vi "PathPlanner_Trajectory25_FindTimeForWaypointRelPos.vi"(9 "WaypointRelPos":dbl, 10 "AllWayPointRelPos":dbl[](array[numeric]), 11 "PathPlannerStates":T1[](array[typedef]) {"ModuleStates"."SWERVE_DRIVE_MODULE_STATE"."Angle"."SIN" format="%13.4f"; "ModuleStates"."SWERVE_DRIVE_MODULE_STATE"."Angle"."COS" format="%13.4f"; "ModuleStates"."SWERVE_DRIVE_MODULE_STATE"."Angle"."VALUE" format="%13.4f"; "ModuleStates"."FieldAngle"."SIN" format="%13.4f"; "ModuleStates"."FieldAngle"."COS" format="%13.4f"; "ModuleStates"."FieldAngle"."VALUE" format="%13.4f"; "ModuleStates"."FieldPos"."Y" format="%14.3f"; "ModuleStates"."FieldPos"."X" format="%14.3f"; "DeltaRot"."SIN" format="%13.4f"; "DeltaRot"."COS" format="%13.4f"; "DeltaRot"."VALUE" format="%13.4f"; "pose"."ROTATION"."SIN" format="%13.4f"; "pose"."ROTATION"."COS" format="%13.4f"; "pose"."ROTATION"."VALUE" format="%13.4f"; "pose"."TRANSLATION"."Y" format="%14.3f"; "pose"."TRANSLATION"."X" format="%14.3f"; "FieldSpeeds"."vOmega" format="%10.3f"; "FieldSpeeds"."vY" format="%10.3f"; "FieldSpeeds"."vX" format="%10.3f"; "Heading"."SIN" format="%13.4f"; "Heading"."COS" format="%13.4f"; "Heading"."VALUE" format="%13.4f"}) -> (3 "Time_Secs":dbl)   [LabVIEW 2019, in "PathPlanner24.lvlib"]
doc: "Find the time (seconds) for a particular waypoint relative position\n\nInputs:\n -- PathPlannerStates -- PathPlanner Trajectory States data cluster\n -- AllWaypointRelPos -- array of double - List of all waypoint relative positions.\n -- WaypointRelPos - double - The waypoint relative positon whose time is desired.\n\nOutputs:\n - Time_Secs - double - The trajectory time for this waypointRelPos."
uses:
  PathPlanner24.lvlib
  TypeDef/PathPlannerTrajectoryState25.ctl
  <vilib>/Rock Robotics/WPI/ThirdParty/JAS_Junk/TrajLib/TypeDef/ROTATION2D.ctl
  TypeDef/PathPlannerPathConstraints.ctl
  <vilib>/Rock Robotics/WPI/ThirdParty/JAS_Junk/TrajLib/TypeDef/CHASSIS_SPEEDS.ctl
  <vilib>/Rock Robotics/WPI/ThirdParty/JAS_Junk/TrajLib/TypeDef/POSE2D.ctl
  <vilib>/Rock Robotics/WPI/ThirdParty/JAS_Junk/TrajLib/TypeDef/TRANSLATION2D.ctl
  TypeDef/PathPlannerSwerveModTrajState.ctl
  <vilib>/Rock Robotics/WPI/ThirdParty/JAS_Junk/TrajLib/TypeDef/SWERVE_DRIVE_MODULE_STATE.ctl
  TypeDef/PathPlannerDriveFeedFwds.ctl
  PathPlanner_GeomUtil_DoubleLerp.vi
  <vilib>/Rock Robotics/WPI/ThirdParty/JAS_Junk/TrajLib/ChassisSpeeds_New.vi
  PathPlanner_DriveFeedFwds_Interpolate.vi
  PathPlanner_GeomUtil_RotationLerp.vi
  <vilib>/Rock Robotics/WPI/ThirdParty/JAS_Junk/TrajLib/MathUtil_Interpolate.vi
  <vilib>/Rock Robotics/WPI/ThirdParty/JAS_Junk/TrajLib/Rotation2d_Minus.vi
  <vilib>/Rock Robotics/WPI/ThirdParty/JAS_Junk/TrajLib/Rotation2d_Times.vi
  <vilib>/Rock Robotics/WPI/ThirdParty/JAS_Junk/TrajLib/Rotation2d_Plus.vi
  <vilib>/Rock Robotics/WPI/ThirdParty/JAS_Junk/TrajLib/MathUtil_Clamp.vi
  <vilib>/Rock Robotics/WPI/ThirdParty/JAS_Junk/TrajLib/Rotation2d_UnaryMinus.vi
  <vilib>/Rock Robotics/WPI/ThirdParty/JAS_Junk/TrajLib/Rotation2d_RotateBy.vi
  <vilib>/Rock Robotics/WPI/ThirdParty/JAS_Junk/TrajLib/Rotation2d_CreateAngle.vi
  <vilib>/Rock Robotics/WPI/ThirdParty/JAS_Junk/TrajLib/Rotation2d_CreateXY.vi
  <vilib>/Rock Robotics/WPI/ThirdParty/JAS_Junk/TrajLib/Util_CalcDist.vi
  <vilib>/gmath/NI_Gmath.lvlib
  <vilib>/Rock Robotics/WPI/ThirdParty/JAS_Junk/TrajLib/Trajectory_Library.lvlib
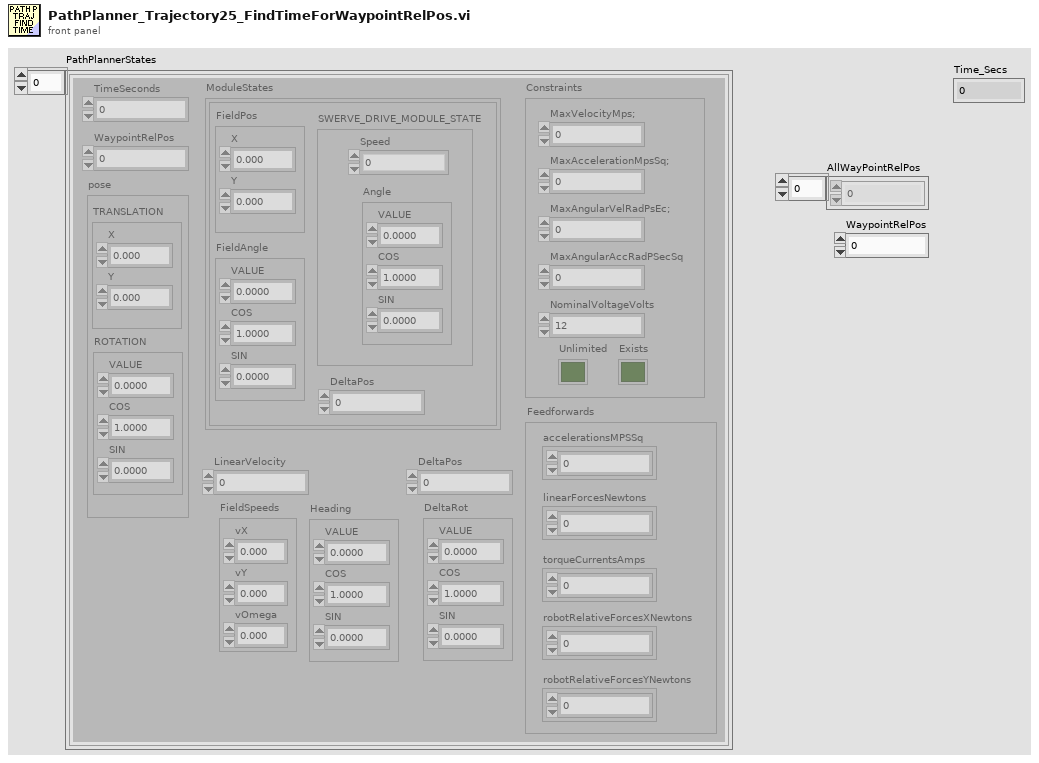
[diagram p1: front panel]
types:
  T1 = typedef "PathPlanner24.lvlib/PathPlannerTrajectoryState25.ctl" = cluster{"TimeSeconds":dbl, "LinearVelocity":dbl, "Heading":T2, "Constraints":T3, "DeltaPos":dbl, "FieldSpeeds":T4, "pose":T5, "DeltaRot":T2, "ModuleStates":T7[], "WaypointRelPos":dbl, "Feedforwards":T9}
  T2 = typedef "Trajectory_Library.lvlib/ROTATION2D.ctl" = cluster{"VALUE":dbl, "COS":dbl, "SIN":dbl}
  T3 = typedef "PathPlanner24.lvlib/PathPlannerPathConstraints.ctl" = cluster{"MaxVelocityMps;":dbl, "MaxAccelerationMpsSq;":dbl, "MaxAngularVelRadPsEc;":dbl, "MaxAngularAccRadPSecSq":dbl, "Exists":bool, "Unlimited":bool, "NominalVoltageVolts":dbl}
  T4 = typedef "Trajectory_Library.lvlib/CHASSIS_SPEEDS.ctl" = cluster{"vX":dbl, "vY":dbl, "vOmega":dbl}
  T5 = typedef "Trajectory_Library.lvlib/POSE2D.ctl" = cluster{"TRANSLATION":T6, "ROTATION":T2}
  T6 = typedef "Trajectory_Library.lvlib/TRANSLATION2D.ctl" = cluster{"X":dbl, "Y":dbl}
  T7 = typedef "PathPlanner24.lvlib/PathPlannerSwerveModTrajState.ctl" = cluster{"FieldPos":T6, "FieldAngle":T2, "DeltaPos":dbl, "SWERVE_DRIVE_MODULE_STATE":T8}
  T8 = typedef "Trajectory_Library.lvlib/SWERVE_DRIVE_MODULE_STATE.ctl" = cluster{"Speed":dbl, "Angle":T2}
  T9 = typedef "PathPlanner24.lvlib/PathPlannerDriveFeedFwds.ctl" = cluster{"accelerationsMPSSq":dbl[], "linearForcesNewtons":dbl[], "torqueCurrentsAmps":dbl[], "robotRelativeForcesXNewtons":dbl[], "robotRelativeForcesYNewtons":dbl[]}
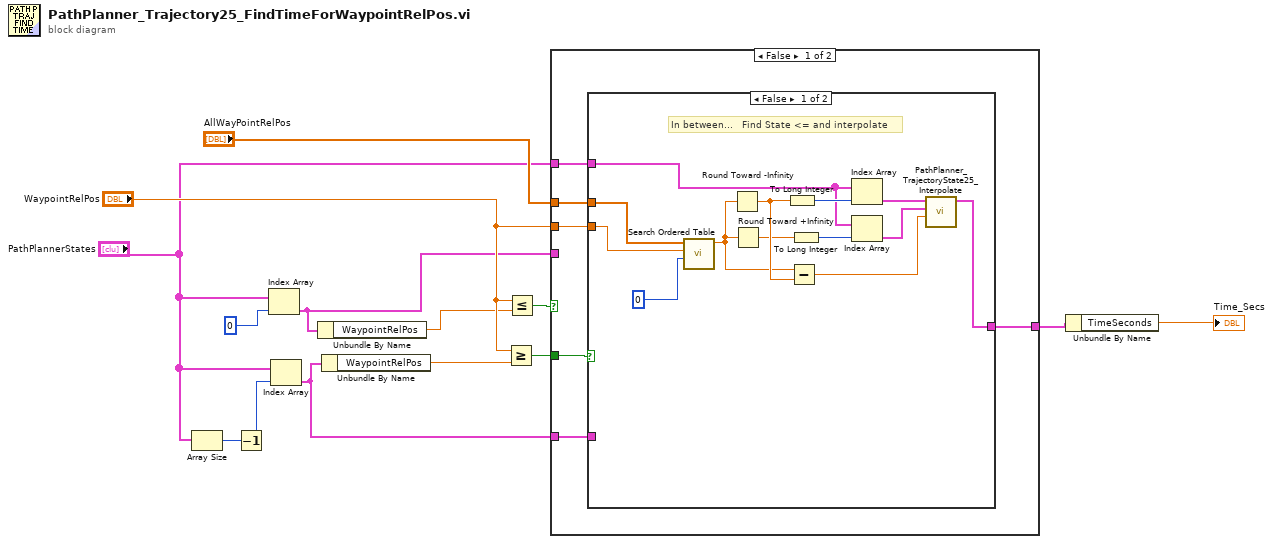
[diagram p0: block diagram]
diagram:
  n1 = Array Size(array="PathPlannerStates") -> (size(s)=w14:i32)
  n2 = Decrement(x=w14) -> (x-1=w7:i32)
  n3 = Index Array(array="PathPlannerStates", index=0) -> (element=w6:T1)
  n4 = Index Array(array="PathPlannerStates", index=w7) -> (element=w3:T1)
  n5 = Unbundle By Name(w6) -> ("WaypointRelPos"=w5:dbl)
  n6 = Unbundle By Name(w3) -> ("WaypointRelPos"=w4:dbl)
  n7 = Greater Or Equal?(x="WaypointRelPos", y=w4) -> (x >= y?=w12:bool)
  n8 = Less Or Equal?(x="WaypointRelPos", y=w5) -> (x <= y?=w13:bool)
  n9 = case shown="False" w13 {
    tunnel: w6 -> [_ w35]
    tunnel: [w18 w35] -> w2
    tunnel: w12 -> [w20 _]
    tunnel: w3 -> [w19 _]
    tunnel: "PathPlannerStates" -> [w17 _]
    tunnel: "AllWayPointRelPos" -> [w16 _]
    tunnel: "WaypointRelPos" -> [w15 _]
    frame False {
      n10 = case shown="False" w20 {
        tunnel: w19 -> [_ w34]
        tunnel: [w21 w34] -> w18
        tunnel: w17 -> [w25 _]
        tunnel: w16 -> [w27 _]
        tunnel: w15 -> [w26 _]
        frame False {
          # "In between...   Find State <= and interpolate"
          n11 = call <vilib>:"Search Ordered Table.vi"("starting index"=0, "x value"=w26, "ordered x array"=w27) -> ("fractional index"=w32:dbl)  [unwired: 8 in]
          n12 = Round Toward -Infinity(1:w32) -> (0:w33:dbl)
          n13 = Round Toward +Infinity(x=w32) -> (ceil(x): smallest int >= x=w31:dbl)
          n14 = To Long Integer(number=w33) -> (32bit integer=w29:i32)
          n15 = Subtract(x=w32, y=w33) -> (x-y=w22:dbl)
          n16 = To Long Integer(number=w31) -> (32bit integer=w30:i32)
          n17 = Index Array(array=w25, index=w29) -> (element=w24:T1)
          n18 = Index Array(array=w25, index=w30) -> (element=w23:T1)
          n19 = call "PathPlanner_TrajectoryState25_Interpolate.vi"("Time"=w22, "end Val"=w23, "in PathPlannerState"=w24) -> ("interpolated PathPlanner State"=w21:T1)  [unwired: 8 in]
        }
        frame True {
          # "WaypointPos > last state, use last."
        }
      }
    }
    frame True {
      # "WaypointRelPos <= First State"
    }
  }
  n20 = Unbundle By Name(w2) -> ("TimeSeconds"=→"Time_Secs":dbl)
